vi "Parse Mode.vi"(8 "error in (no error)":errorcluster, 9 "SPI_Mode In":T1, 10 "index":i32, 11 "Mode":string) -> (0 "error out":errorcluster, 3 "SPI_Mode":T1)   [LabVIEW 2018, in "Config_Read_SPI.lvclass"]
uses:
  Config_Read_SPI.lvclass
  SPI_Mode.ctl
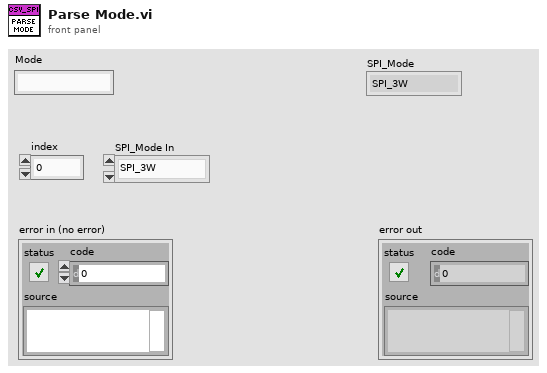
[diagram p1: front panel]
types:
  T1 = typedef "Config_Read_SPI.lvclass/SPI_Mode.ctl" = enum16{"SPI_3W", "SPI_4W"}
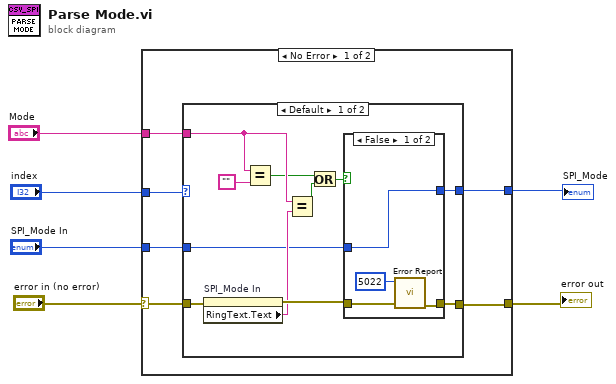
[diagram p0: block diagram]
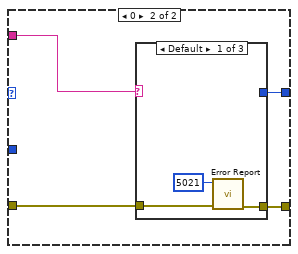
[diagram p3: hidden frame]
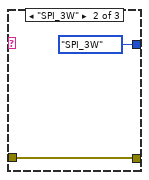
[diagram p4: hidden frame]
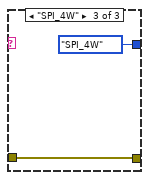
[diagram p5: hidden frame]
diagram:
  n1 = case shown="No Error" "error in (no error)" {
    selector: "error in (no error)" -> [w10 w42]
    tunnel: [w9 w42] -> w5
    tunnel: "Mode" -> [w11 _]
    tunnel: "index" -> [w12 _]
    tunnel: [w8 w41] -> w2
    tunnel: "SPI_Mode In" -> [w7 w41]
    frame No Error {
      n2 = case shown="Default" w12 {
        tunnel: w11 -> [w17 w31]
        tunnel: w10 -> [w21 w33]
        tunnel: [w23 w32] -> w9
        tunnel: [w22 w30] -> w8
        tunnel: w7 -> [w18 _]
        frame Default {
          n3 = property on="SPI_Mode In" class="Enum (strict)"(error in=w21) -> (error out=w20:errorcluster, "RingText.Text"=w19:string)  [unwired: 1 in, 1 out]
          n4 = Equal?(x=w17, y="") -> (x = y?=w14:bool)
          n5 = Equal?(x=w17, y=w19) -> (x = y?=w15:bool)
          n6 = Or(x=w14, y=w15) -> (x .or. y?=w13:bool)
          n7 = case shown="False" w13 {
            tunnel: w20 -> [w27 w28]
            tunnel: [w26 w28] -> w23
            tunnel: [w24 w29] -> w22
            tunnel: w18 -> [w24 w29]
            frame False {
              n8 = call "Error Report.vi"("error in (no error)"=w27, "Error Code"=i16 5022) -> ("error out"=w26:errorcluster)  [unwired: 9 in]
            }
            frame True {
            }
          }
        }
        frame 0 {
          n9 = case shown="Default" w31 {
            tunnel: w33 -> [w36 w38 w40]
            tunnel: [w35 w38 w40] -> w32
            tunnel: [_ SPI_Mode."SPI_3W" ("SPI_Mode 2") SPI_Mode."SPI_4W" ("SPI_Mode 2")] -> w30
            frame Default {
              n10 = call "Error Report.vi"("error in (no error)"=w36, "Error Code"=i16 5021) -> ("error out"=w35:errorcluster)  [unwired: 9 in]
            }
            frame "SPI_3W" {
            }
            frame "SPI_4W" {
            }
          }
        }
      }
    }
    frame Error {
    }
  }
  "error out" <- w5
  "SPI_Mode" <- w2
